vi "Compute Gate-IRF Array.vi"(8 "Error In":errorcluster, 9 "Gate & Decay Parameters":T1 {"A" format="%#_4g"; "s" format="%#_4g"; "sF" format="%#_4g"; "sR" format="%#_4g"; "t_i" format="%#_4g"; "t_0" format="%#_4g"; "tau" format="%#_4g"; "T" format="%#_4g"; "W" format="%#_4g"}, 11 "X":dbl[](array[numeric])) -> (0 "Error Out":errorcluster, 3 "IRF/Gate Array":dbl[](array[numeric]))   [LabVIEW 2019]
uses:
  Gate & Decay Parameters.ctl
  Gate Type.ctl
  IRF Model.ctl
  Graphs/XY Graph/XY Plot Data.ctl
  <vilib>/Utility/error.llb/Error Cluster From Error Code.vi
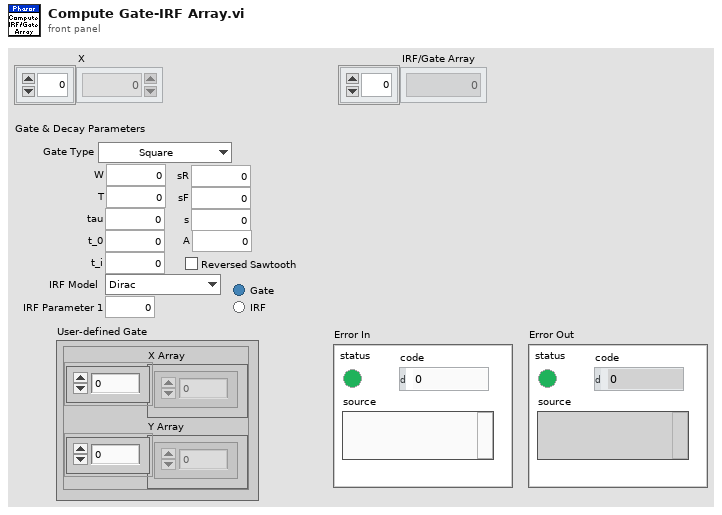
[diagram p1: front panel]
types:
  T1 = typedef "Gate & Decay Parameters.ctl" = cluster{"W":dbl, "T":dbl, "tau":dbl, "t_0":dbl, "Gate Type":T2, "t_i":dbl, "sR":dbl, "sF":dbl, "s":dbl, "Reversed Sawtooth":bool, "IRF Model":T3, "IRF Parameter 1":dbl, "User-defined Gate":T4, "Type of User-defined Function":enum32{"Gate", "IRF"}, "A":dbl}
  T2 = typedef "Gate Type.ctl" = enum16{"Square", "Finite Edge Square", "Finite Edge, Tilted Top Square", "Triangle", "Sawtooth", "User-defined"}
  T3 = typedef "IRF Model.ctl" = enum16{"Dirac", "Exponential"}
  T4 = typedef "XY Plot Data.ctl" = cluster{"X Array":dbl[], "Y Array":dbl[]}
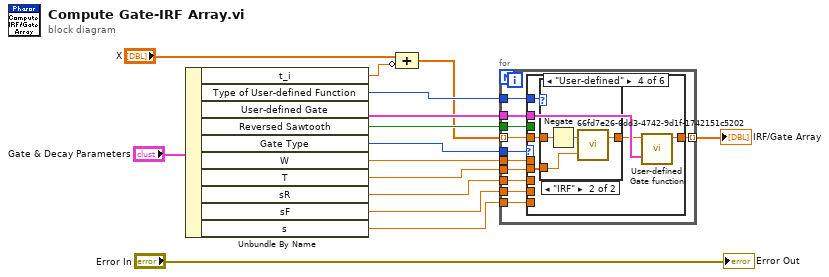
[diagram p0: block diagram]
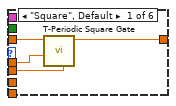
[diagram p2: hidden frame]
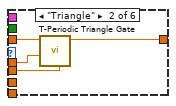
[diagram p3: hidden frame]
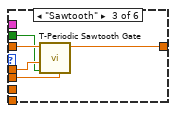
[diagram p4: hidden frame]
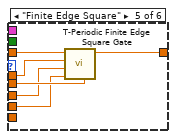
[diagram p6: hidden frame]
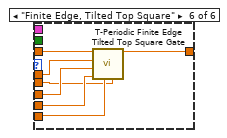
[diagram p7: hidden frame]
diagram:
  n1 = Unbundle By Name("Gate & Decay Parameters") -> ("t_i"=w1:dbl, "Type of User-defined Function"=w9:enum32{"Gate", "IRF"}, "User-defined Gate"=w10:T4, "Reversed Sawtooth"=w11:bool, "Gate Type"=w2:T2, "W"=w3:dbl, "T"=w4:dbl, "sR"=w7:dbl, "sF"=w6:dbl, "s"=w5:dbl)
  n2 = Compound Arithmetic op=ADD("X", invert w1) -> (w8:dbl[])
  n3 = for {
    tunnel: w4 -> [w17]
    tunnel: w8 -> [w26] mode=indexing
    tunnel: w2 -> [w25]
    tunnel: [w24] -> w13 mode=indexing
    tunnel: w3 -> [w23]
    tunnel: w7 -> [w22]
    tunnel: w6 -> [w21]
    tunnel: w5 -> [w20]
    tunnel: w11 -> [w19]
    tunnel: w10 -> [w18]
    tunnel: w9 -> [w16]
    n4 = case shown="\"User-defined\"" w25 {
      tunnel: w23 -> [w29 w34 w38 _ w54 w61]
      tunnel: w26 -> [w30 w33 w39 w45 w56 w63]
      tunnel: [w28 w32 w37 w44 w55 w62] -> w24
      tunnel: w22 -> [_ _ _ _ w52 w60]
      tunnel: w21 -> [_ _ _ _ w51 w59]
      tunnel: w20 -> [_ _ _ _ _ w58]
      tunnel: w19 -> [_ _ w36 _ _ _]
      tunnel: w18 -> [_ _ _ w43 _ _]
      tunnel: w17 -> [w27 w31 w35 w42 w53 w57]
      tunnel: w16 -> [_ _ _ w40 _ _]
      frame "Square", Default {
        n5 = call "T-Periodic Square Gate.vi"("Period T"=w27, "W"=w29, "t"=w30) -> ("Square(t)"=w28:dbl)  [unwired: 8 in]
      }
      frame "Triangle" {
        n6 = call "T-Periodic Triangle Gate.vi"("Period T"=w31, "W"=w34, "t"=w33) -> ("Triangle(t)"=w32:dbl)  [unwired: 8 in]
      }
      frame "Sawtooth" {
        n7 = call "T-Periodic Sawtooth Gate.vi"("Period T"=w35, "Reversed?"=w36, "W"=w38, "t"=w39) -> ("Sawtooth(t)"=w37:dbl)  [unwired: 7 in]
      }
      frame "User-defined" {
        n8 = case shown="\"IRF\"" w40 {
          tunnel: w45 -> [w46 w50]
          tunnel: w42 -> [_ w48]
          tunnel: [w46 w47] -> w41
          frame "Gate", Default {
          }
          frame "IRF" {
            n9 = Negate(x=w50) -> (-x=w49:dbl)
            n10 = call "66fd7e26-6dd3-4742-9d1f-1742151c5202.vi"("y"=w48, "x"=w49) -> ("x - E(x/y)y"=w47:dbl)  [unwired: 1 out]
          }
        }
        n11 = call "User-defined Gate function.vi"("User-defined Gate"=w43, "t"=w41) -> ("User-defined Gate(t)"=w44:dbl)  [unwired: 8 in, 1 out]
      }
      frame "Finite Edge Square" {
        n12 = call "T-Periodic Finite Edge Square Gate.vi"("Period T"=w53, "s_F"=w51, "s_R"=w52, "W"=w54, "t"=w56) -> ("Finite Edge Square(t)"=w55:dbl)  [unwired: 6 in]
      }
      frame "Finite Edge, Tilted Top Square" {
        n13 = call "T-Periodic Finite Edge Tilted Top Square Gate.vi"("Period T"=w57, "slope"=w58, "s_F"=w59, "s_R"=w60, "W"=w61, "t"=w63) -> ("Finite Edge Square(t)"=w62:dbl)  [unwired: 5 in]
      }
    }
  }
  "IRF/Gate Array" <- w13
  "Error Out" <- "Error In"
